vi "Mech on_off.vi"(6 "Peripherals in":T1, 8 "error in (no error)":errorcluster, 10 "Motors":bool=TRUE) -> (0 "error out":errorcluster, 2 "auto off log":string, 4 "Peripherals out":T1)   [LabVIEW 2014, in "AISAS Mech.lvclass"]
uses:
  AISAS Mech.lvclass
  Controls/peripherals.ctl
  AISAS Mech.lvclass/AISAS Mech.ctl
  motor/AISAS motor.lvclass/AISAS motor.ctl
  motor/AISAS motor.lvclass
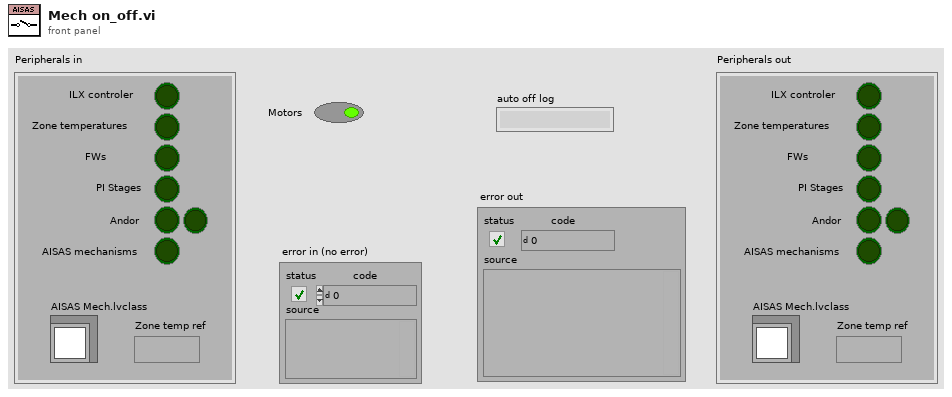
[diagram p1: front panel]
types:
  T1 = typedef "peripherals.ctl" = cluster{"ILX controler":bool, "Zone temperatures":bool, "Andor":bool, "Andor 2":bool, "PI Stages":bool, "AISAS mechanisms":bool, "AISAS Mech.lvclass":refnum<class "AISAS Mech.lvclass">, "Zone temp ref":variant, "FWs":bool}
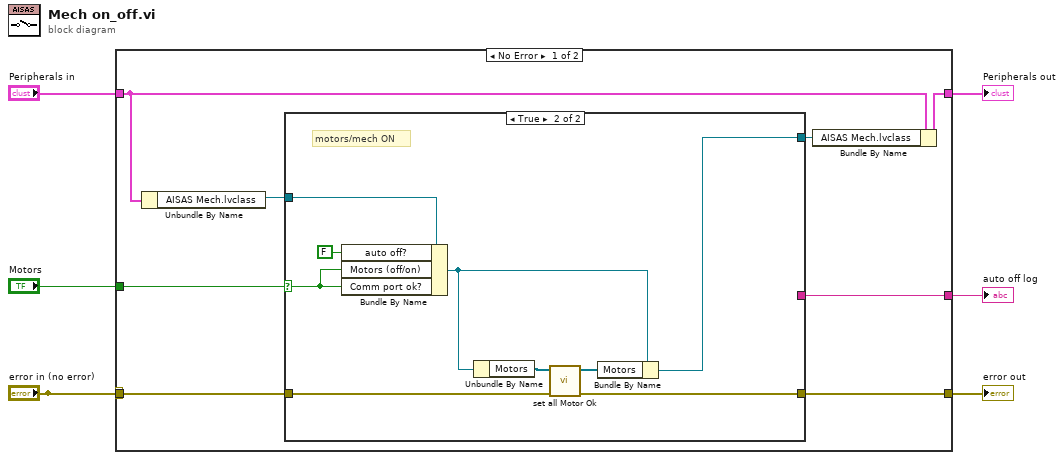
[diagram p0: block diagram]
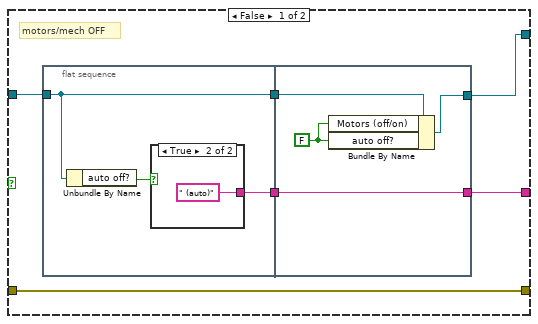
[diagram p2: hidden frame]
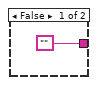
[diagram p3: hidden frame]
diagram:
  n1 = case shown="No Error" "error in (no error)" {
    selector: "error in (no error)" -> [_ w40]
    tunnel: [w14 w40] -> w6
    tunnel: [w13 _] -> w5
    tunnel: "error in (no error)" -> [w12 _]
    tunnel: "Motors" -> [w11 _]
    tunnel: "Peripherals in" -> [w8 w39]
    tunnel: [w7 w39] -> w1
    frame No Error {
      n2 = Unbundle By Name(w8) -> ("AISAS Mech.lvclass"=w10:refnum<class "AISAS Mech.lvclass">)
      n3 = case shown="True" w11 {
        selector: w11 -> [_ w38]
        tunnel: [w16 w31] -> w14
        tunnel: [w20 _] -> w13
        tunnel: w12 -> [w16 w34]
        tunnel: w10 -> [w17 w36]
        tunnel: [w15 w30] -> w9
        frame False {
          # "motors/mech OFF"
          n4 = flat-sequence {
            tunnel: w17 -> [w21]
            tunnel: [w23] -> w19
            tunnel: [w21] -> w18
            tunnel: [w29] -> w20
            tunnel: w19 -> [w29]
            tunnel: w18 -> [w28]
            tunnel: [w26] -> w15
            frame #0 {
              n5 = Unbundle By Name(w21) -> ("auto off?"=w22:bool)
              n6 = case shown="True" w22 {
                tunnel: ["" " (auto)" ("Sync response")] -> w23
                frame False {
                }
                frame True {
                }
              }
            }
            frame #1 {
              w27 = FALSE ("Motors (off/on)")
              n7 = Bundle By Name(cluster=w28, "Motors (off/on)"=w27, "auto off?"=w27) -> (w26:refnum<class "AISAS Mech.lvclass">)
            }
          }
        }
        frame True {
          # "motors/mech ON"
          n8 = Bundle By Name(cluster=w36, "auto off?"=FALSE, "Motors (off/on)"=w38, "Comm port ok?"=w38) -> (w33:refnum<class "AISAS Mech.lvclass">)
          n9 = Unbundle By Name(w33) -> ("Motors"=w35:refnum<class "AISAS motor.lvclass">[])
          n10 = call "set all Motor Ok.vi"("error in (no error)"=w34, "AISAS Motors"=w35) -> ("error out"=w31:errorcluster, "AISAS Motors out"=w32:refnum<class "AISAS motor.lvclass">[])  [unwired: 8 in]
          n11 = Bundle By Name(cluster=w33, "Motors"=w32) -> (w30:refnum<class "AISAS Mech.lvclass">)
        }
      }
      n12 = Bundle By Name(cluster=w8, "AISAS Mech.lvclass"=w9) -> (w7:T1)
    }
    frame Error {
    }
  }
  "error out" <- w6
  "auto off log" <- w5
  "Peripherals out" <- w1
